vi "drivetrain_reset_encoders.vi"() -> (1 "Avg Velocity (Ft/Sec)":dbl, 2 "Velocity (in/sec)":cluster{"Left":dbl, "Right":dbl}, 3 "Distance (in)":cluster{"Left":dbl, "Right":dbl})   [LabVIEW 2011]
panel:
  out "error out 2":errorcluster
  out "error out":errorcluster
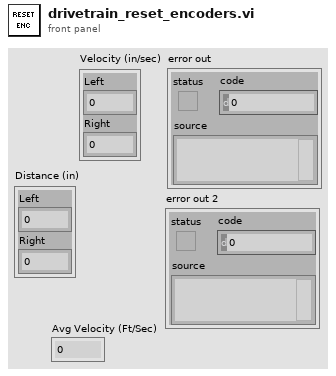
[diagram p1: front panel]
types:
  T1 = typedef "WPI_EncoderDevRef.ctl" = cluster{"DevStatus":errorcluster, "EncoderIndex":T2, "CounterIndex":T3, "DistancePerCount":dbl, "Decoding Type":T4}
  T2 = typedef "FPGA_EncoderIdx.ctl" = enum8{"Enc 0", "Enc 1", "Enc 2", "Enc 3", "Invalid"}
  T3 = typedef "FPGA_CounterCtrSystemIndex.ctl" = enum8{"Ctr 0", "Ctr 1", "Ctr 2", "Ctr 3", "Ctr 4", "Ctr 5", "Ctr 6", "Ctr 7", "Invalid"}
  T4 = typedef "WPI_EncoderType.ctl" = enum16{"1x", "2x", "4x"}
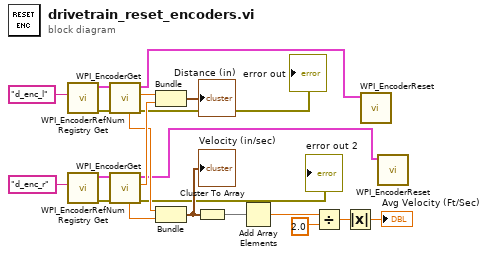
[diagram p0: block diagram]
diagram:
  n1 = call <vilib>:"WPI_EncoderRefNum Registry Get.vi"("refnum name"="d_enc_l") -> ("error out"=w6:errorcluster, "EncoderDevRef"=w19:T1)  [unwired: 9 in]
  n2 = call <vilib>:"WPI_EncoderRefNum Registry Get.vi"("refnum name"="d_enc_r") -> ("error out"=w5:errorcluster, "EncoderDevRef"=w18:T1)  [unwired: 9 in]
  n3 = call <vilib>:"WPI_EncoderGet.vi"("error in (no error)"=w6, "EncoderDevRef"=w19) -> ("error out"=→"error out":errorcluster, "Distance"=w16:dbl, "EncoderDevRef"=w2:T1, "Rate"=w14:dbl)  [unwired: 4 in, 2 out]
  n4 = call <vilib>:"WPI_EncoderGet.vi"("error in (no error)"=w5, "EncoderDevRef"=w18) -> ("error out"=→"error out 2":errorcluster, "Distance"=w15:dbl, "EncoderDevRef"=w1:T1, "Rate"=w13:dbl)  [unwired: 4 in, 2 out]
  n5 = Bundle("Distance"=w16, "Distance"=w15) -> (→"Distance (in)":cluster{"Distance":dbl, "Distance":dbl})  [unwired: 1 in]
  n6 = Bundle("Rate"=w14, "Rate"=w13) -> (w12:cluster{"Rate":dbl, "Rate":dbl})  [unwired: 1 in]
  "Velocity (in/sec)" <- w12
  n7 = Cluster To Array(cluster=w12) -> (array=w11:dbl[])
  n8 = Add Array Elements(numeric array=w11) -> (sum=w10:dbl)
  n9 = Divide(x=w10, y=2.0) -> (x/y=w8:dbl)
  n10 = Absolute Value(x=w8) -> (abs(x)=→"Avg Velocity (Ft/Sec)":dbl)
  n11 = call <vilib>:"WPI_EncoderReset.vi"("EncoderDevRef"=w2) -> ()  [unwired: 9 in, 2 out]
  n12 = call <vilib>:"WPI_EncoderReset.vi"("EncoderDevRef"=w1) -> ()  [unwired: 9 in, 2 out]
